vi "Init.vi"(8 "error in (no error)":errorcluster, 10 "Muted":bool, 11 "Input Name":string) -> (0 "error out":errorcluster, 3 "SetInputMute out":refnum<class "SetInputMute.lvclass">)   [LabVIEW 2020, in "obs-websocket.lvlib" / "SetInputMute.lvclass"]
uses:
  SetInputMute.lvclass
  SetInputMute.lvclass/SetInputMute.ctl
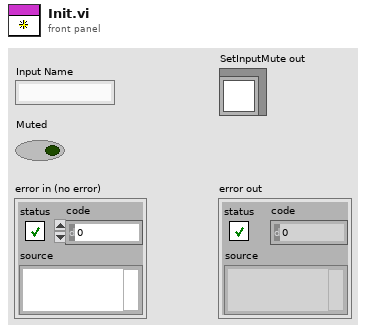
[diagram p1: front panel]
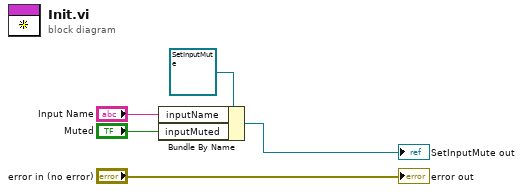
[diagram p0: block diagram]
diagram:
  n1 = Bundle By Name(cluster=refnum<class "SetInputMute.lvclass"> refnum ("SetInputMute in"), "inputName"="Input Name", "inputMuted"="Muted") -> (→"SetInputMute out":refnum<class "SetInputMute.lvclass">)
  "error out" <- "error in (no error)"
